vi "Stop.vi"(0 "reference in":refnum<class "Slide.lvclass">, 5 "error in (no error)":errorcluster) -> (14 "reference out":refnum<class "Slide.lvclass">, 19 "error out":errorcluster)   [LabVIEW 2013, in "Slide.lvclass"]
uses:
  Slide.lvclass
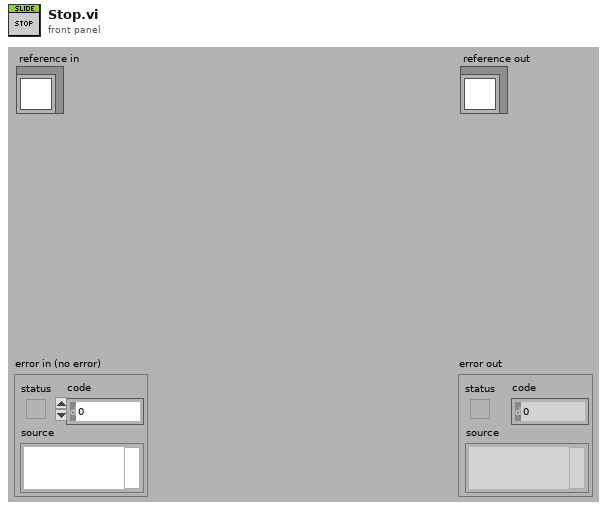
[diagram p1: front panel]
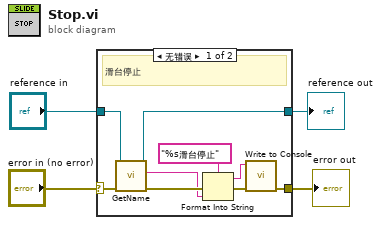
[diagram p0: block diagram]
diagram:
  n1 = case shown="无错误" "error in (no error)" {
    selector: "error in (no error)" -> [w13 w15]
    tunnel: [w7 w15] -> w3
    tunnel: [w5 w14] -> w1
    tunnel: "reference in" -> [w6 w14]
    frame No Error {
      # "滑台停止"
      n2 = call-dynamic "GetName.vi"("error in (no error)"=w13, "reference in"=w6) -> ("error out"=w11:errorcluster, "Name"=w10:string, "reference out"=w5:refnum<class "Slide.lvclass">)  [unwired: 7 in]
      n3 = Format Into String(format string="%s滑台停止" ("Input"), error in=w11, w10) -> (resulting string=w8:string, error out=w9:errorcluster)  [unwired: 1 in]
      n4 = call "Write to Console.vi"("error in (no error)"=w9, "Input"=w8) -> ("error out"=w7:errorcluster)  [unwired: 9 in]
    }
    frame Error {
    }
  }
  "error out" <- w3
  "reference out" <- w1
